vi "Get Window Image.vi"(8 "error in (no error)":errorcluster, 11 "window refnum in":T2) -> (0 "error out":errorcluster, 2 "image data":T1, 3 "window refnum out":T2)   [LabVIEW 2020, in "MacroAssert.lvlib" / "Win Util.lvlib"]
doc: "This VI will use window refnum in to get the name of a window. The name of a window is simply the text appearing in the title bar of the window. If the title bar of the window is not shown, the name of the window will be a NULL string."
uses:
  Win Util.lvlib
  Window Refnum.ctl
  <vilib>/picture/picture.llb/imagedata.ctl
  System.Drawing
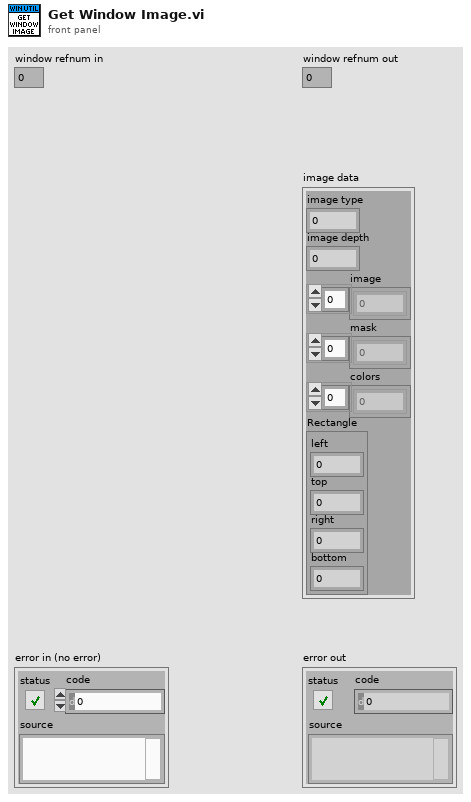
[diagram p1: front panel]
types:
  T1 = typedef "imagedata.ctl" = cluster{"image type":i32, "image depth":i32, "image":u8[], "mask":u8[], "colors":u32[], "Rectangle":cluster{"left":i16, "top":i16, "right":i16, "bottom":i16}}
  T2 = typedef "MacroAssert.lvlib/Win Util.lvlib/Window Refnum.ctl" = u64
  T3 = cluster{"left":i16, "top":i16, "right":i16, "bottom":i16}
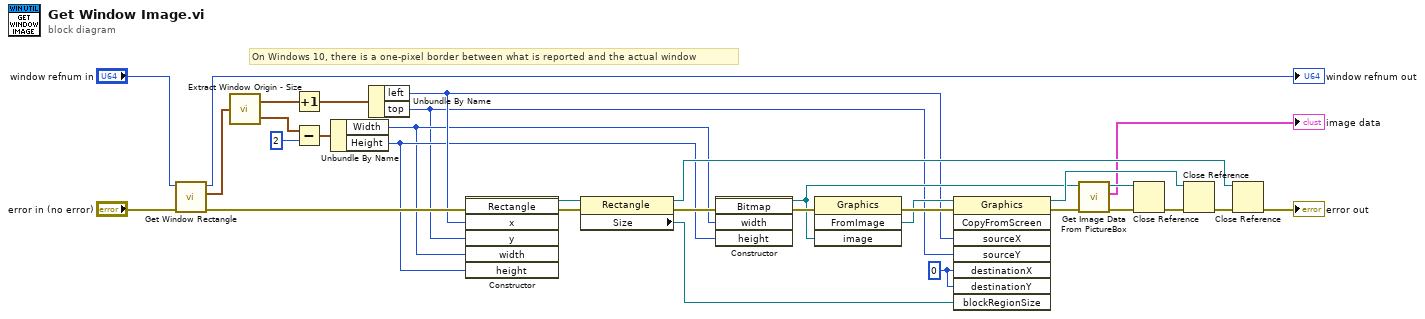
[diagram p0: block diagram]
diagram:
  w5 = 0 ("destinationX")
  # "On Windows 10, there is a one-pixel border between what is reported and the actual window"
  n1 = call "Get Window Rectangle.vi"("error in (no error)"="error in (no error)", "window refnum (NaWR)"="window refnum in") -> ("error out"=w26:errorcluster, "window rect"=w9:T3, "window refnum out"=→"window refnum out":T2)  [unwired: 7 in]
  n2 = call "Extract Window Origin - Size.vi"("window rect"=w9) -> ("window origin"=w8:cluster{"left":i16, "top":i16}, "window size"=w10:cluster{"Width":i16, "Height":i16})
  n3 = Increment(x=w8) -> (x+1=w3:cluster{"left":i16, "top":i16})
  n4 = Subtract(x=w10, y=i16 2) -> (x-y=w2:cluster{"Width":i16, "Height":i16})
  n5 = Unbundle By Name(w2) -> ("Width"=w11:i16, "Height"=w12:i16)
  n6 = Unbundle By Name(w3) -> ("left"=w13:i16, "top"=w4:i16)
  n7 = constructor class="Rectangle"(error in=w26, "x"=w13, "y"=w4, "width"=w11, "height"=w12) -> (reference out=w17:refnum<k24>, error out=w25:errorcluster)  [unwired: 2 in, 5 out]
  n8 = property class="Rectangle"(reference=w17, error in=w25) -> (reference out=w18:refnum<k24>, error out=w23:errorcluster, "Size"=w21:refnum<k24>)
  n9 = constructor class="Bitmap"(error in=w23, "width"=w11, "height"=w12) -> (reference out=w16:refnum<k24>, error out=w31:errorcluster)  [unwired: 2 in, 3 out]
  n10 = invoke class="Graphics" method="FromImage"(error in=w31, "image"=w16) -> (error out=w24:errorcluster, "FromImage"=w15:refnum<k24>)  [unwired: 2 in, 2 out]
  n11 = invoke class="Graphics" method="CopyFromScreen"(reference=w15, error in=w24, "sourceX"=w13, "sourceY"=w4, "destinationX"=w5, "destinationY"=w5, "blockRegionSize"=w21) -> (reference out=w19:refnum<k24>, error out=w32:errorcluster)  [unwired: 1 in, 6 out]
  n12 = call "Get Image Data From PictureBox.vi"("error in (no error)"=w32, "Image"=w16) -> ("error out"=w30:errorcluster, "Image Data"=→"image data":T1, "Image Out"=w20:refnum<k24>)  [unwired: 7 in]
  n13 = Close Reference(reference=w20, error in (no error)=w30) -> (error out=w29:errorcluster)
  n14 = Close Reference(reference=w19, error in (no error)=w29) -> (error out=w28:errorcluster)
  n15 = Close Reference(reference=w18, error in (no error)=w28) -> (error out=→"error out":errorcluster)
